vi "Read Channels array.vi"(8 "error in (no error)":errorcluster, 11 "AutoExp in":refnum<class "AutoExp.lvclass">) -> (0 "error out":errorcluster, 2 "Channels array":refnum<class "Channel.lvclass">[](array[class]), 3 "AutoExp out":refnum<class "AutoExp.lvclass">)   [LabVIEW 2018, in "AutoExp.lvclass"]
uses:
  AutoExp.lvclass
  Channel/Channel.lvclass
  AutoExp.lvclass/AutoExp.ctl
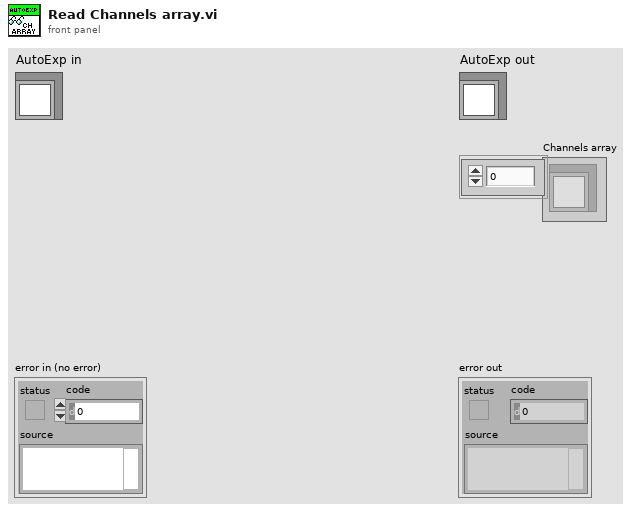
[diagram p1: front panel]
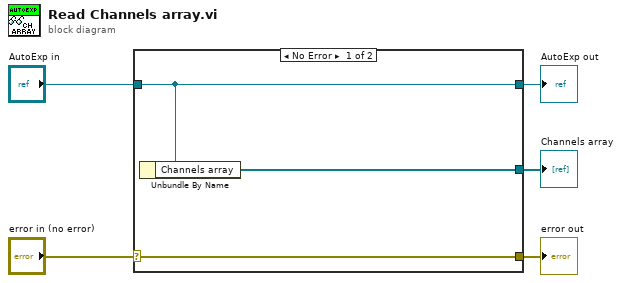
[diagram p0: block diagram]
diagram:
  n1 = case shown="No Error" "error in (no error)" {
    selector: "error in (no error)" -> [w8 w9]
    tunnel: [w8 w9] -> w4
    tunnel: [w7 w10] -> w2
    tunnel: "AutoExp in" -> [w7 w10]
    tunnel: [w6 _] -> w1
    frame No Error {
      n2 = Unbundle By Name(w7) -> ("Channels array"=w6:refnum<class "Channel.lvclass">[])
    }
    frame Error {
    }
  }
  "error out" <- w4
  "AutoExp out" <- w2
  "Channels array" <- w1
